vi "DivBinning.vi"(7 "Settings.number of cam":dbl, 10 "offset":dbl, 11 "spec cluster 3":cluster{"dp [MeV/C]":dbl[], dbl[]}[](graph)) -> (1 "spec cluster":cluster{"xi used":dbl[], "yi":dbl[]}(graph), 2 "divergence":waveform(dbl), 5 "time:div":u32)   [LabVIEW 2011]
uses:
  NI_Gmath.lvlib
  NI_AALBase.lvlib
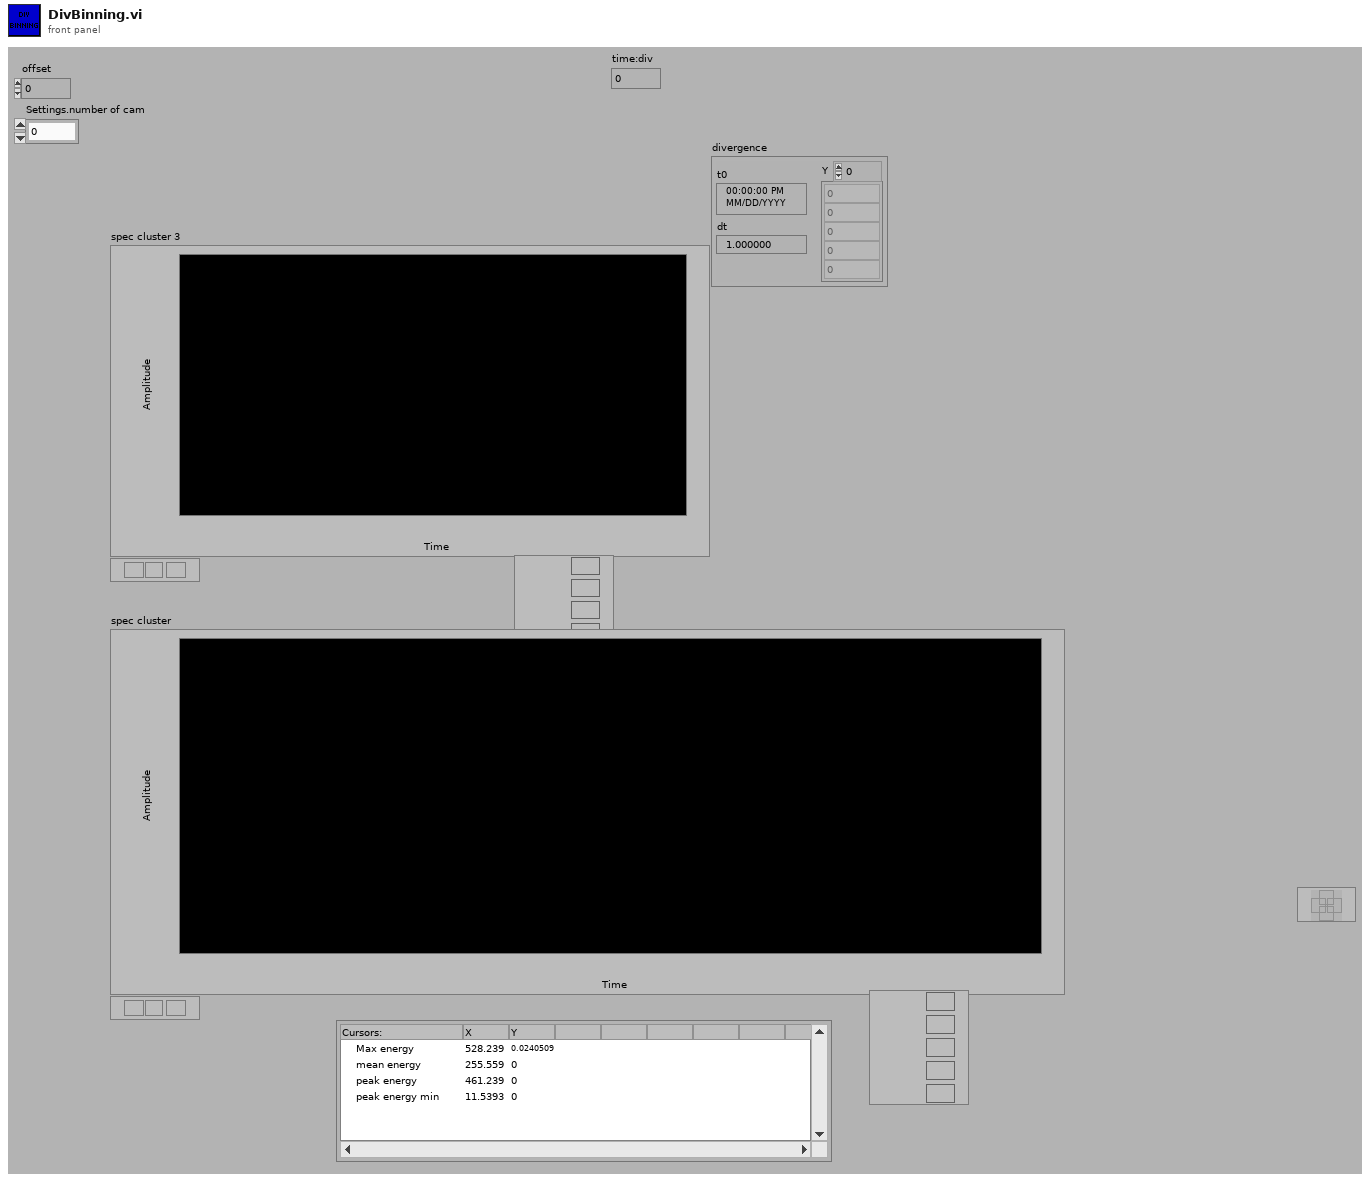
[diagram p1: front panel]
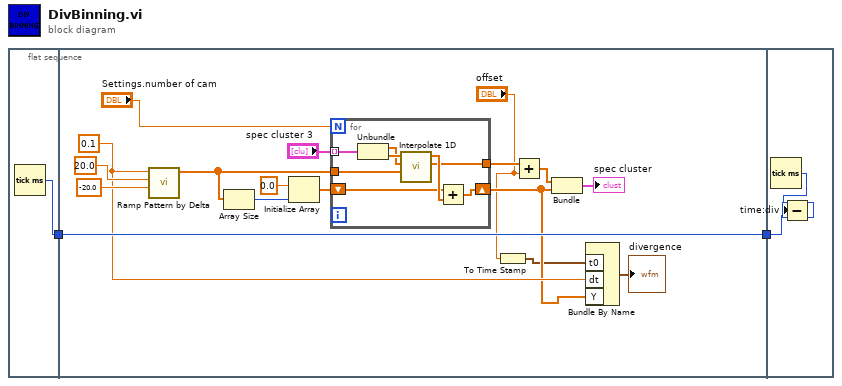
[diagram p0: block diagram]
diagram:
  n1 = flat-sequence {
    tunnel: [w3] -> w2
    tunnel: w2 -> [w11]
    tunnel: [w11] -> w1
    tunnel: w1 -> [w30]
    frame #0 {
      n2 = Tick Count (ms)() -> (millisecond timer value=w3:u32)
    }
    frame #1 {
      w9 = 0.1 ("delta")
      n3 = call "Ramp Pattern by Delta.vi"("start"=-20.0, "end"=20.0, "delta"=w9) -> ("Ramp Pattern"=w16:dbl[])  [unwired: 6 in, 2 out]
      n4 = Array Size(array=w16) -> (size(s)=w15:i32)
      n5 = Initialize Array(0.0 ("delta"), w15) -> (w14:dbl[])
      n6 = for {
        N: "Settings.number of cam" -> [_]
        tunnel: "spec cluster 3" -> [w28] mode=indexing
        tunnel: w16 -> [w25]
        shift-right: [w22] -> w7
        shift-left: w14 -> [w23]
        tunnel: [w21] -> w12
        n7 = Unbundle(w28) -> ("dp [MeV/C]"=w26:dbl[], w27:dbl[])
        n8 = call "Interpolate 1D.vi"("xi"=w25, "X"=w26, "Y"=w27) -> ("xi used"=w21:dbl[], "yi"=w24:dbl[])  [unwired: 6 in, 1 out]
        n9 = Add(x=w23, y=w24) -> (x+y=w22:dbl[])
      }
      n10 = To Time Stamp(1:"offset") -> (0:w5:timestamp)
      n11 = Add(x=w12, y="offset") -> (x+y=w8:dbl[])
      n12 = Bundle(w8, w7) -> (→"spec cluster":cluster{dbl[], dbl[]})  [unwired: 1 in]
      n13 = Bundle By Name("t0"=w5, "dt"=w9, "Y"=w7) -> (→"divergence":waveform(dbl))  [unwired: 1 in]
    }
    frame #2 {
      n14 = Tick Count (ms)() -> (millisecond timer value=w31:u32)
      n15 = Subtract(x=w31, y=w30) -> (x-y=→"time:div":u32)
    }
  }
